vi "Open-lasing-file.vi"(8 "error in (no error)":errorcluster, 10 "File index":i32, 11 "Object ref in":T1) -> (0 "error out":errorcluster, 1 "Succes?":bool, 3 "Object ref out":T1)   [LabVIEW 2013, in "SLMControl.lvlib" / "SC-Main.lvclass"]
uses:
  SC-Main.lvclass
  Object-reference.ctl
  SC-Main.lvclass/SC-Main.ctl
  Read Status.vi
  Read Lasing files.vi
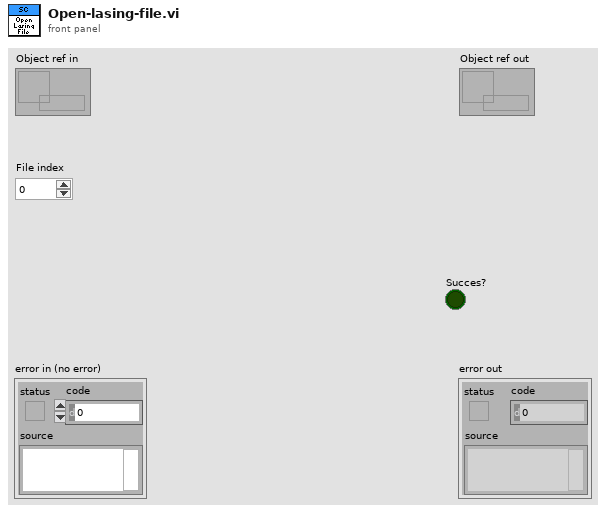
[diagram p1: front panel]
types:
  T1 = typedef "SLMControl.lvlib/SC-Main.lvclass/Object-reference.ctl" = refnum<data-value>
  T2 = typedef "SLMControl.lvlib/SC-Main.lvclass/Client-status.ctl" = enum16{"Idle", "Initialized", "Configured", "Activated", "Started", "Paused", "Stopped", "Reset", "Error", "Exited"}
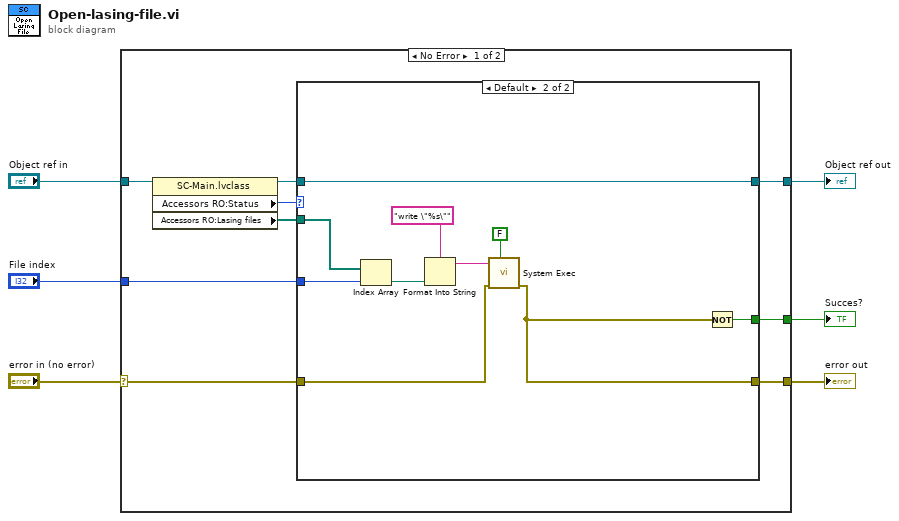
[diagram p0: block diagram]
diagram:
  n1 = case shown="No Error" "error in (no error)" {
    selector: "error in (no error)" -> [w15 w29]
    tunnel: [w12 w29] -> w5
    tunnel: [w11 w28] -> w3
    tunnel: "Object ref in" -> [w14 w28]
    tunnel: [w8 _] -> w2
    tunnel: "File index" -> [w7 _]
    frame No Error {
      n2 = property class="SC-Main.lvclass"(reference=w14) -> (reference out=w13:T1, "Accessors RO:Status"=w10:T2, "Accessors RO:Lasing files"=w9:path[])  [unwired: 1 in, 1 out]
      n3 = case shown="Default" w10 {
        tunnel: w15 -> [w16 w24]
        tunnel: w13 -> [w17 w27]
        tunnel: [w16 w18] -> w12
        tunnel: [w17 w27] -> w11
        tunnel: w9 -> [_ w25]
        tunnel: [_ w19] -> w8
        tunnel: w7 -> [_ w26]
        frame "Started", "Paused" {
        }
        frame Default {
          n4 = Index Array(array=w25, index=w26) -> (element=w22:path)
          n5 = Format Into String(format string="write \"%s\"", w22) -> (resulting string=w20:string)  [unwired: 2 in, 1 out]
          n6 = call <vilib>:"System Exec.vi"("wait until completion? (T)"=FALSE, "error in (no error)"=w24, "command line"=w20) -> ("error out"=w18:errorcluster)  [unwired: 5 in, 3 out]
          n7 = Not(x=w18) -> (.not. x?=w19:bool)
        }
      }
    }
    frame Error {
    }
  }
  "error out" <- w5
  "Object ref out" <- w3
  "Succes?" <- w2
